vi "Read Last Series.vi"(11 "Result in":refnum<class "Result.lvclass">) -> (2 "Series":refnum<class "Series.lvclass">, 3 "Result out":refnum<class "Result.lvclass">)   [LabVIEW 2018, in "InfluxDB Client.lvlib" / "Result.lvclass"]
uses:
  Result.lvclass
  Series/Series.lvclass
  Result.lvclass/Result.ctl
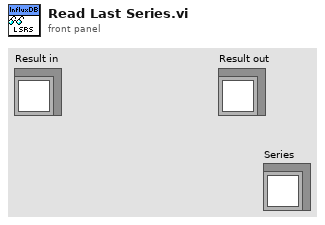
[diagram p1: front panel]
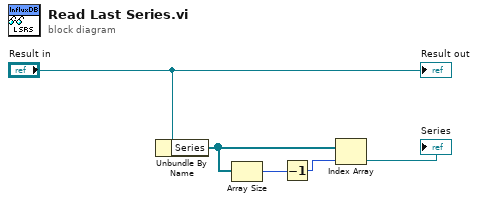
[diagram p0: block diagram]
diagram:
  n1 = Unbundle By Name("Result in") -> ("Series"=w4:refnum<class "Series.lvclass">[])
  n2 = Array Size(array=w4) -> (size(s)=w3:i32)
  n3 = Decrement(x=w3) -> (x-1=w2:i32)
  n4 = Index Array(array=w4, index=w2) -> (element=→"Series":refnum<class "Series.lvclass">)
  "Result out" <- "Result in"
